vi "Autonomous Independent.vi"() -> ()   [LabVIEW 2015]
doc: "This VI is called when autonomous begins, and will automatically be terminated when autonomous ends. You can carry out timed or sensor driven robot movement independently without needing to return to the caller."
uses:
  <vilib>/Analysis/coordinate.llb/2D Cartesian Coordinate Rotation (Scalar).vi
  <vilib>/Analysis/coordinate.llb/2D Cartesian Coordinate Shift (Array).vi
  <vilib>/Rock Robotics/WPI/Utilities/WPI_GetSetVariantRefNum.vi
  <vilib>/Rock Robotics/Network Tables/SD Write Numeric Array.vi
  <vilib>/addons/control/pid/pid.llb/PID (DBL).vi
  <vilib>/Rock Robotics/WPI/RobotDrive/WPI_RobotDriveMecanumDrive_Polar.vi
  <vilib>/Analysis/NI_AALPro.lvlib
  <vilib>/addons/control/pid/NI_PID_pid.lvlib
  <vilib>/Rock Robotics/Network Tables/SD Read Number.vi
  <vilib>/Rock Robotics/WPI/RobotDrive/WPI_RobotDriveMecanumDrive_Cartesian.vi
panel:
  out "Y Out":dbl[](array[numeric])
  out "X Out":dbl[](array[numeric])
  out "Current Movement, for debugging":T1 {"Z Joystick Value" scale=-1.0..1.0; "Y Joystick Value" scale=1.0..-1.0; "X Joystick Value" scale=-1.0..1.0}
  in  "Array of robot movements":T2(array[cluster]) {"Z Joystick Value" scale=-1.0..1.0; "Y Joystick Value" scale=1.0..-1.0; "X Joystick Value" scale=-1.0..1.0}
  # "Be sure to right-click and choose Data Operations>>Make Current Value default if you want to save the array values with the VI"
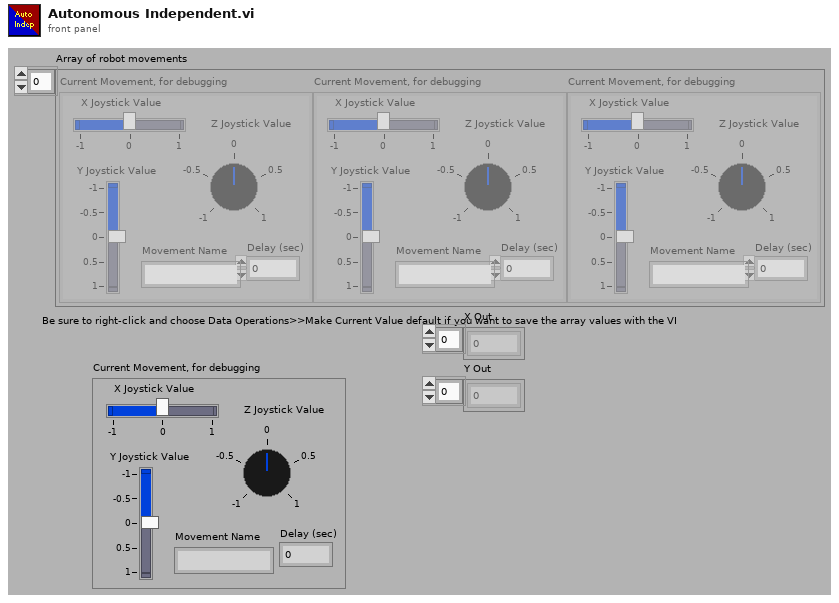
[diagram p1: front panel]
types:
  T1 = cluster{"X Joystick Value":dbl, "Y Joystick Value":dbl, "Z Joystick Value":dbl, "Delay (sec)":dbl, "Movement Name":string}
  T2 = cluster{"X Joystick Value":dbl, "Y Joystick Value":dbl, "Z Joystick Value":dbl, "Delay (sec)":dbl, "Movement Name":string}[]
  T3 = enum16{"Bin In", "Move Back", "Move Right", "Push Forward", "Stop"}
  T4 = typedef "WPI_JoystickDevRef.ctl" = cluster{"Device":T5}
  T5 = typedef "WPI_JoystickDeviceEnum.ctl" = enum16{"USB 0", "USB 1", "USB 2", "USB 3", "USB 4", "USB 5"}
  T6 = enum16{"Bin In", "Bin Up", "Tote In", "Move Sideways", "Advance", "Turn", "Dive Forward"}
  T7 = cluster{"proportional gain (Kc)":dbl, "integral time (Ti, min)":dbl, "derivative time (Td, min)":dbl}
  T8 = typedef "WPI_RobotDriveDevRef.ctl" = cluster{"DevStatus":errorcluster, "Motors[]":T9[], "Square Inputs":bool, "Max Output":dbl}
  T9 = typedef "WPI_MotorControlDeviceRef.ctl" = cluster{"DeviceStatus":errorcluster, "Type":T10, "PWM":cluster{"PWM Channel":T11, "DeadBand":T12}, "CAN":cluster{"Device Number":u8, "Control Mode":T13, "Semaphore":T14, "Max Vout":dbl, "TalonSRX Control Mode":T15}, "Invert":bool}
  T10 = typedef "WPI_MotorControlType.ctl" = enum16{"PWM", "CAN", "CANTalonSRX"}
  T11 = typedef "FPGA_DIOPWMChannel.ctl" = enum8{"PWM 0", "PWM 1", "PWM 2", "PWM 3", "PWM 4", "PWM 5", "PWM 6", "PWM 7", "PWM 8", "PWM 9", "PWM MXP 0", "PWM MXP 1", "PWM MXP 2", "PWM MXP 3", "PWM MXP 4", "PWM MXP 5", "PWM MXP 6", "PWM MXP 7", "PWM MXP 8", "PWM MXP 9", "Invalid"}
  T12 = typedef "WPI_PWMDeadband.ctl" = cluster{"Name":string, "maxPositivePwm":i32, "minPositivePwm":i32, "centerPwm":i32, "maxNegativePwm":i32, "minNegativePwm":i32, "angularRange":u16}
  T13 = typedef "WPI_CANJaguar_ControlMode.ctl" = enum8{"Percent VBus", "Current", "Speed", "Position", "Voltage"}
  T14 = typedef "Semaphore RefNum" = refnum<k1>
  T15 = typedef "WPI_CANTalonSRX_APIControlMode.ctl" = enum8{"Percent VBus", "Speed", "Position", "Slave", "Unchanged / Invalid", "Voltage Compensation", "Current", "Motion Profile"}
  T16 = typedef "WPI_GyroDevRef.ctl" = cluster{"DevStatus":errorcluster, "Analog Channel":T17, "Offset":dbl, "Gain (VoltsPerDegree/Second)":dbl, "Gyro Type":enum16{"Analog", "XRS450"}, "Handle":i32, "SPI Bus":T18, "Device Found":bool, "Sample Rate":dbl, "Calibrate On Open":bool}
  T17 = typedef "FPGA_AIChannel.ctl" = enum8{"AI 0", "AI 1", "AI 2", "AI 3", "AI MXP 0", "AI MXP 1", "AI MXP 2", "AI MXP 3", "Invalid"}
  T18 = typedef "spi_bus.ctl" = enum16{"SPI On-Board, CS0", "SPI On-Board, CS1", "SPI On-Board, CS2", "SPI On-Board, CS3", "SPI MXP", "Invalid"}
  T19 = typedef "WPI_DigitalInputDevRef.ctl" = cluster{"DevStatus":errorcluster, "DIO Channel":T20}
  T20 = typedef "FPGA_DIOChannel.ctl" = enum8{"DIO 0", "DIO 1", "DIO 2", "DIO 3", "DIO 4", "DIO 5", "DIO 6", "DIO 7", "DIO 8", "DIO 9", "DIO MXP 0", "DIO MXP 1", "DIO MXP 2", "DIO MXP 3", "DIO MXP 4", "DIO MXP 5", "DIO MXP 6", "DIO MXP 7", "DIO MXP 8", "DIO MXP 9", "DIO MXP 10", "DIO MXP 11", "DIO MXP 12", "DIO MXP 13", "DIO MXP 14", "DIO MXP 15", "Invalid"}
  T21 = typedef "WPI_AccelerometerDevRef.ctl" = cluster{"DevStatus":errorcluster, "Scaling":T22, "Analog Channels":T23, "I2C Bus":T24, "SPI Bus":T18, "Accel Range":T25, "ADXL Axes":T26, "Handle":i32, "Device Address":u8, "Accel Type":enum16{"Analog", "ADXL345 I2C", "ADXL345 SPI", "Internal", "ADXL362 SPI"}}
  T22 = typedef "WPI_AccelerometerScaling.ctl" = cluster{"Gain (VoltsPerG)":dbl, "Center Voltage":dbl}
  T23 = typedef "WPI_AccelerometerAnalogChannels.ctl" = cluster{"X-Axis":T17, "Y-Axis":T17, "Z-Axis":T17}
  T24 = typedef "i2c_bus.ctl" = enum16{"I2C On-Board", "I2C MXP", "Invalid"}
  T25 = typedef "ADXL345 Range.ctl" = u8
  T26 = typedef "WPI_AccelerometerADXL345 Axes.ctl" = cluster{"X-Axis":bool, "Y-Axis":bool, "Z-Axis":bool}
  T27 = cluster{"X-Axis":dbl, "Y-Axis":dbl, "Z-Axis":dbl}
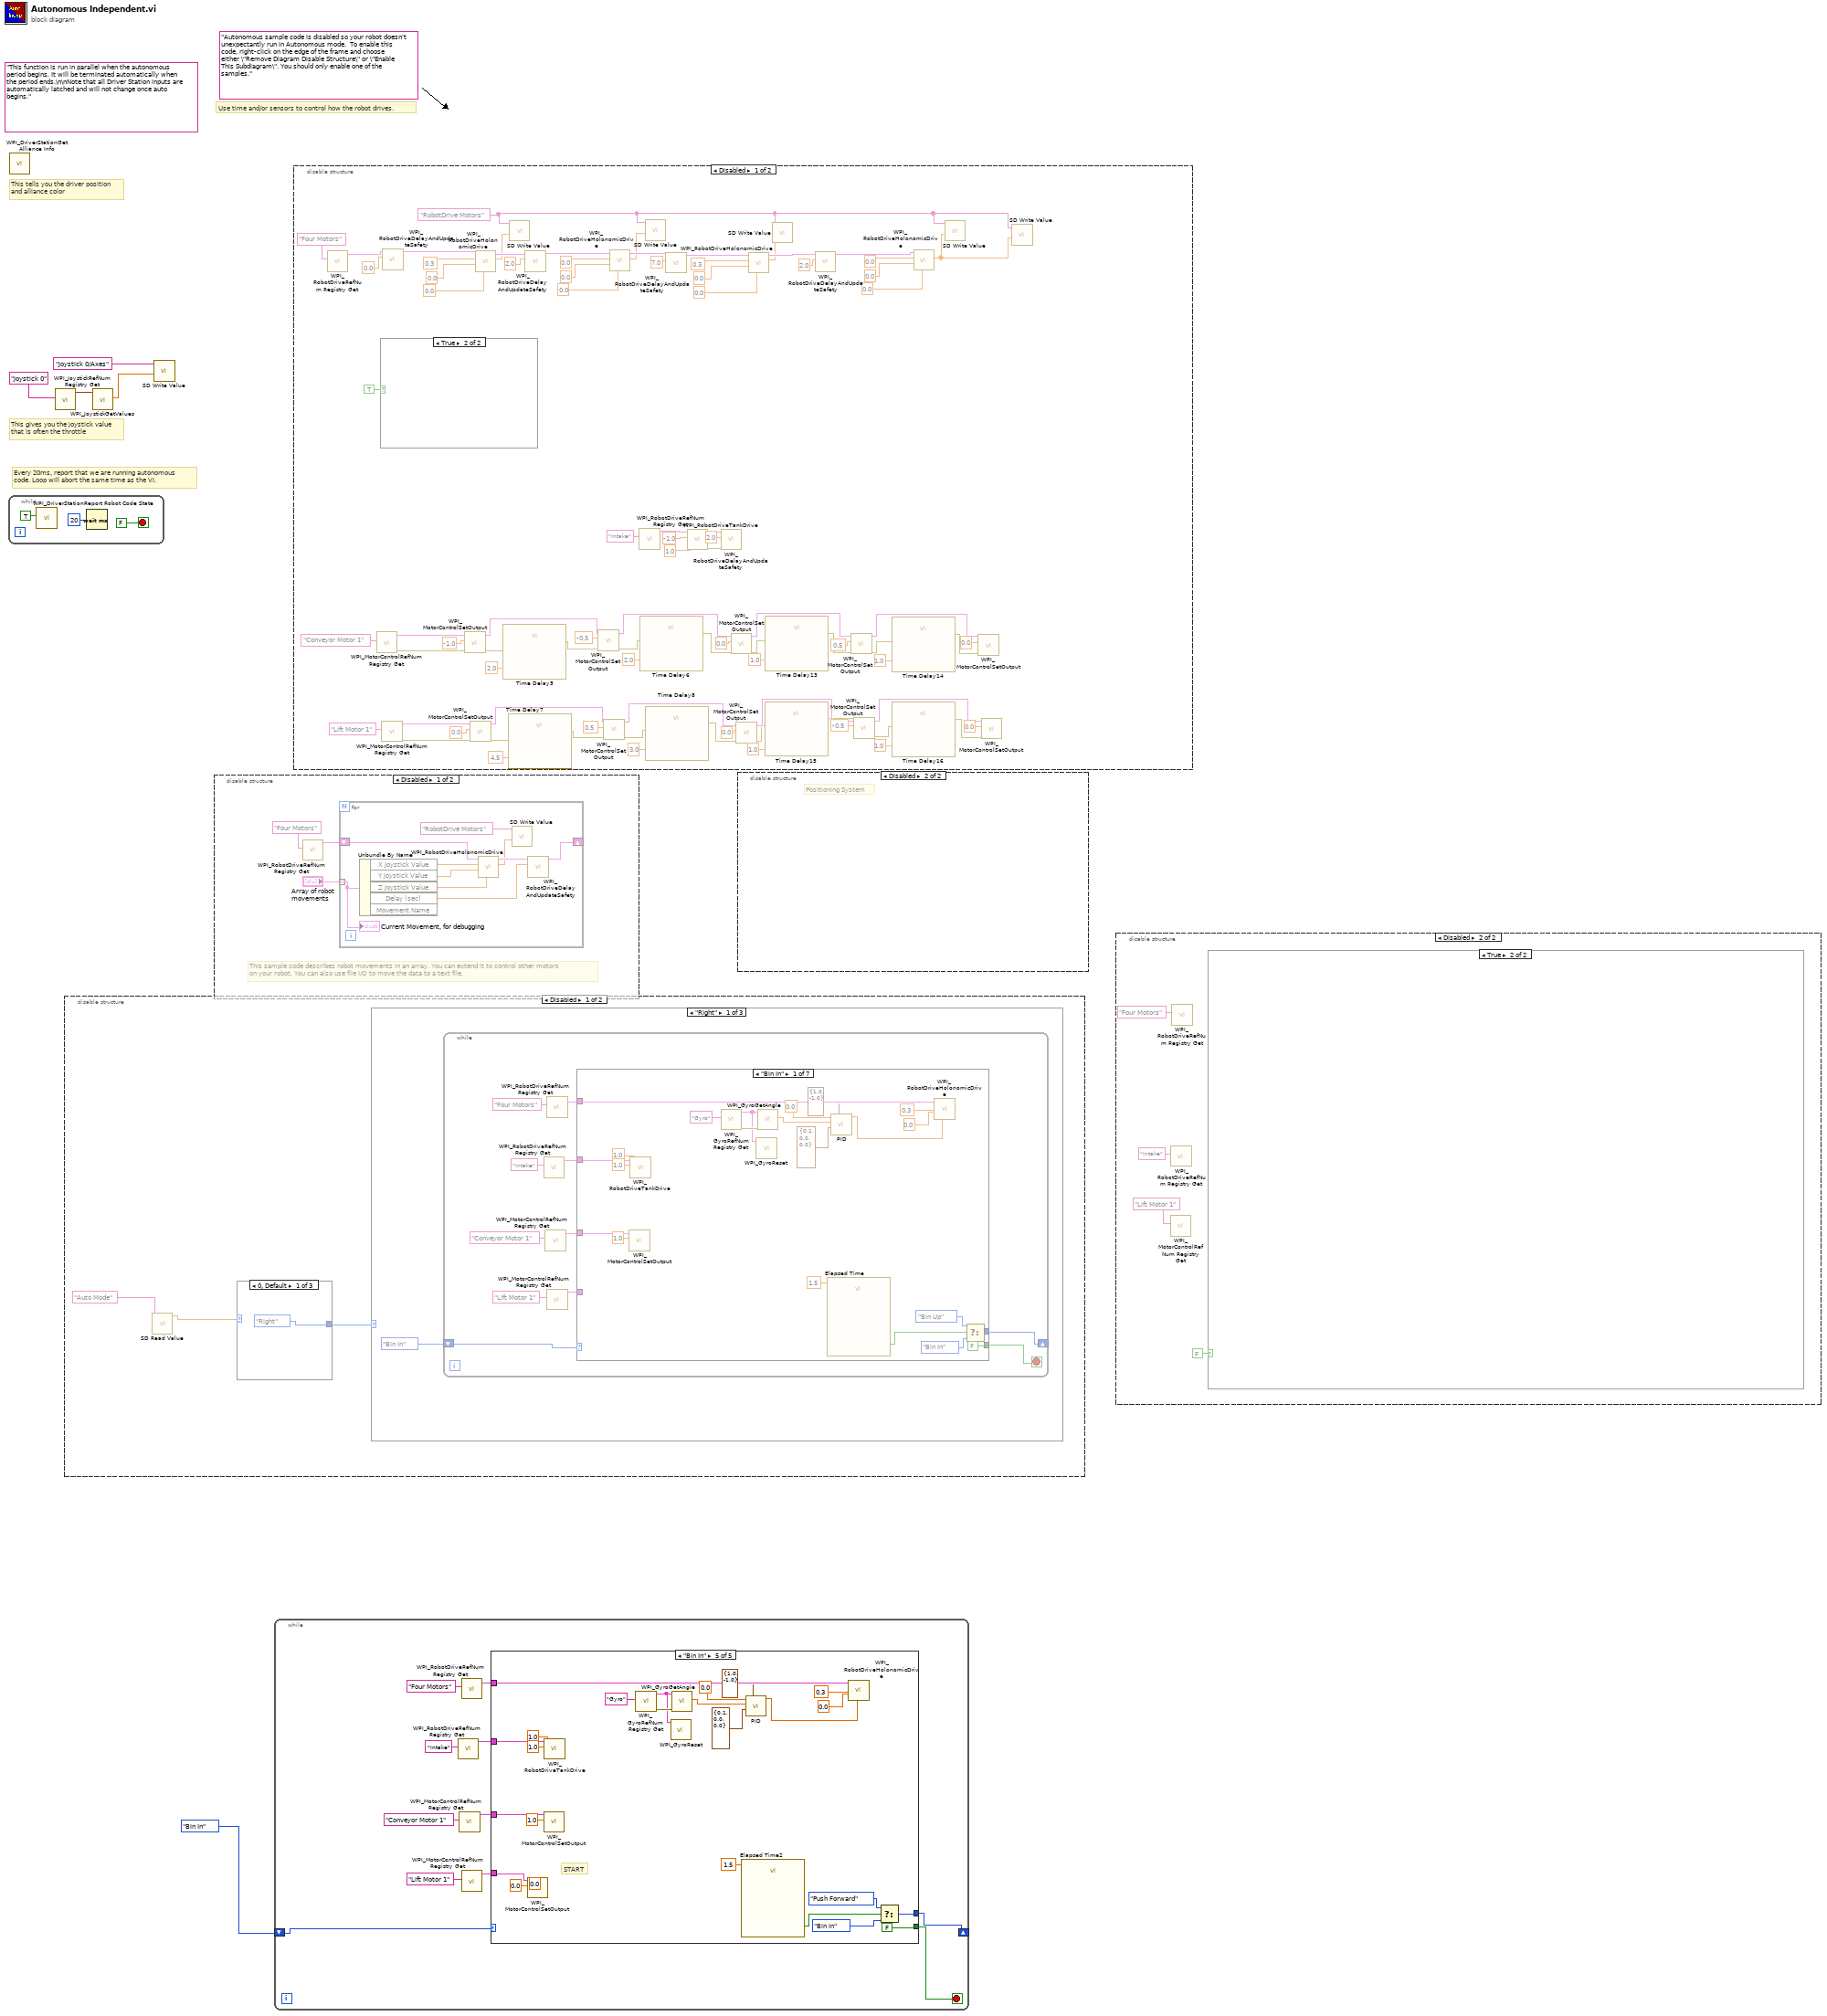
[diagram p0: block diagram]
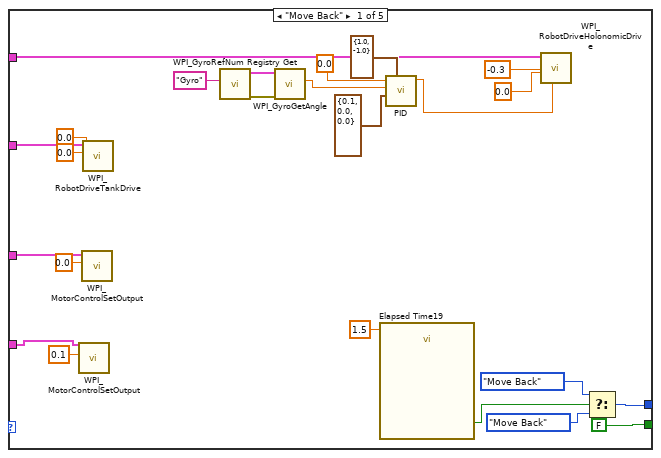
[diagram p2: hidden frame]
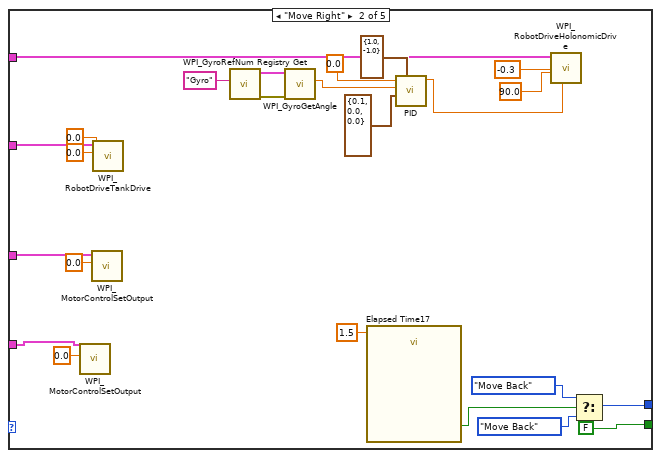
[diagram p3: hidden frame]
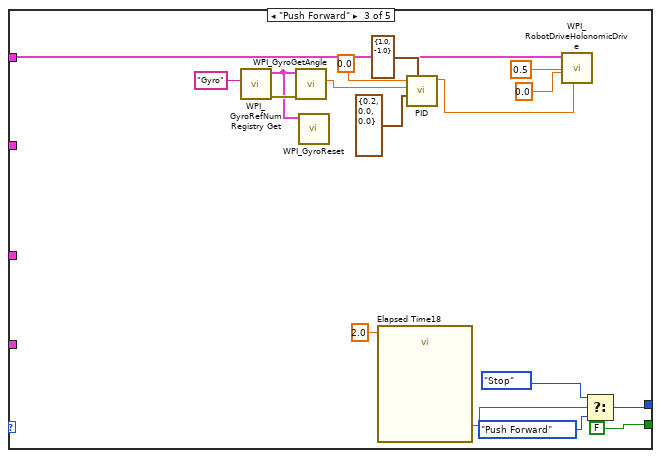
[diagram p4: hidden frame]
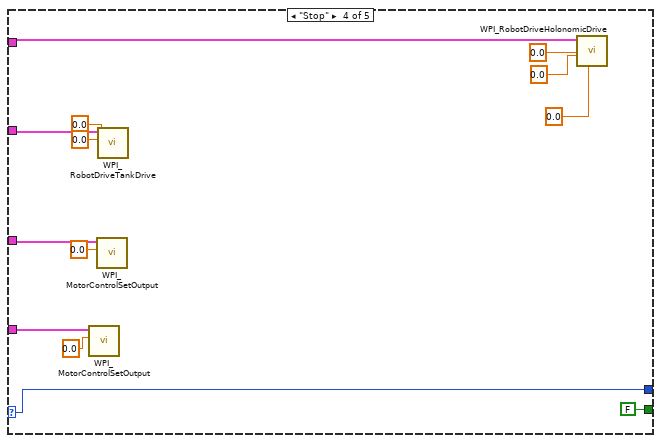
[diagram p5: hidden frame]
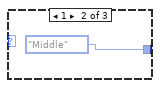
[diagram p6: hidden frame]
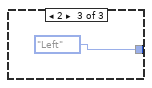
[diagram p7: hidden frame]
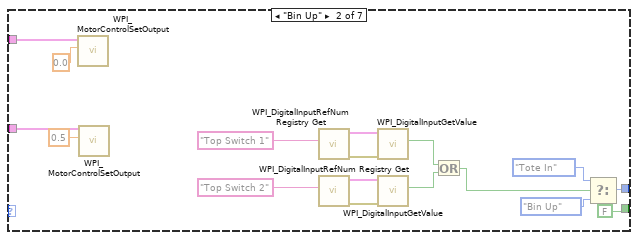
[diagram p8: hidden frame]
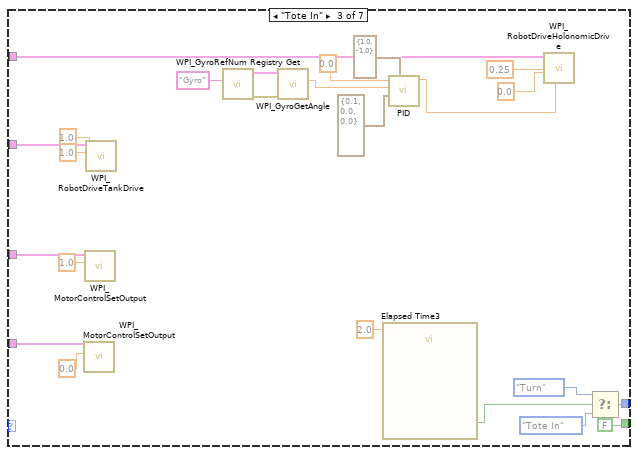
[diagram p9: hidden frame]
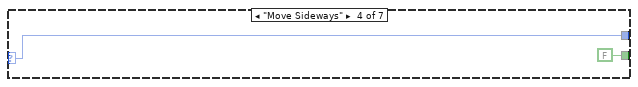
[diagram p10: hidden frame]
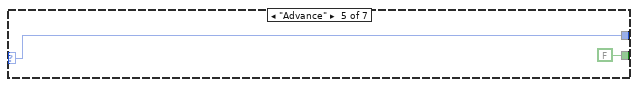
[diagram p11: hidden frame]
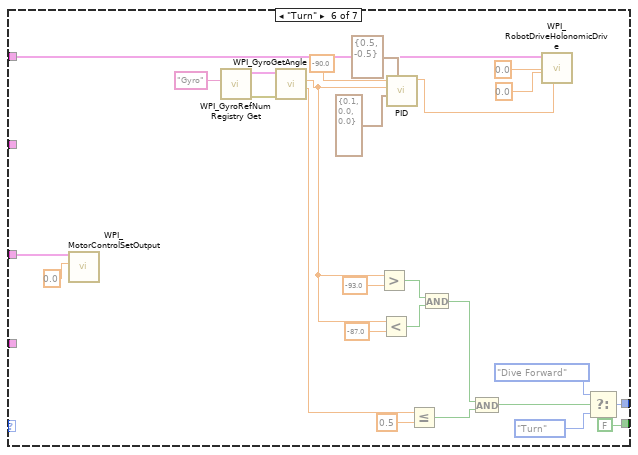
[diagram p12: hidden frame]
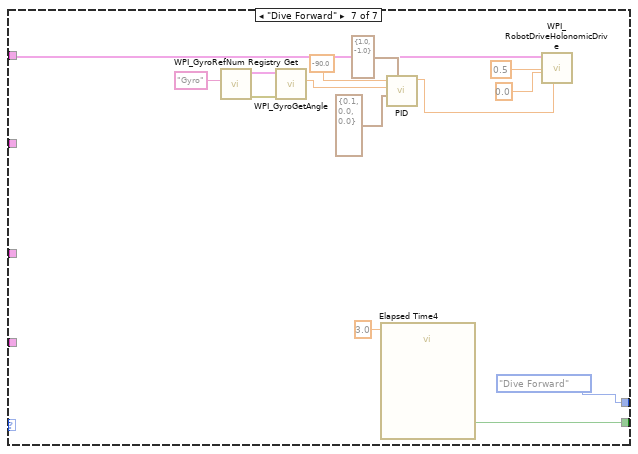
[diagram p13: hidden frame]
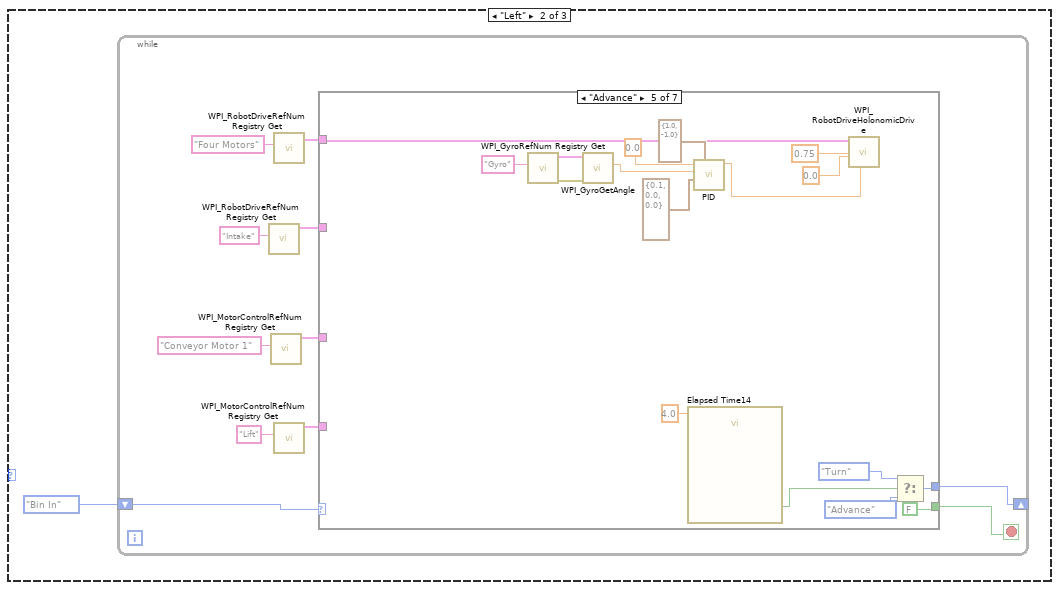
[diagram p14: hidden frame]
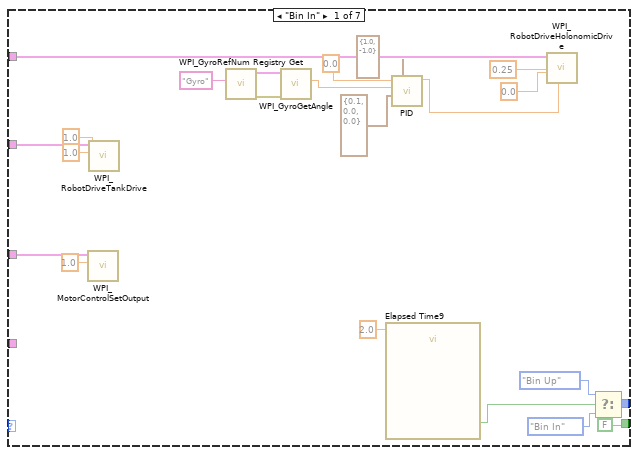
[diagram p15: hidden frame]
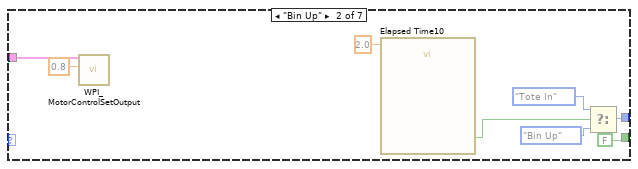
[diagram p16: hidden frame]
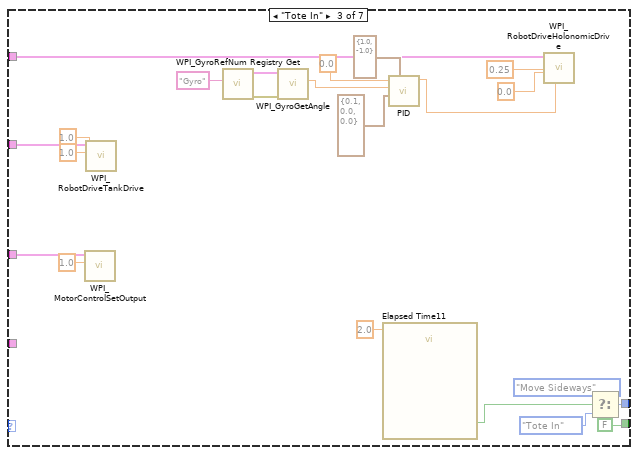
[diagram p17: hidden frame]
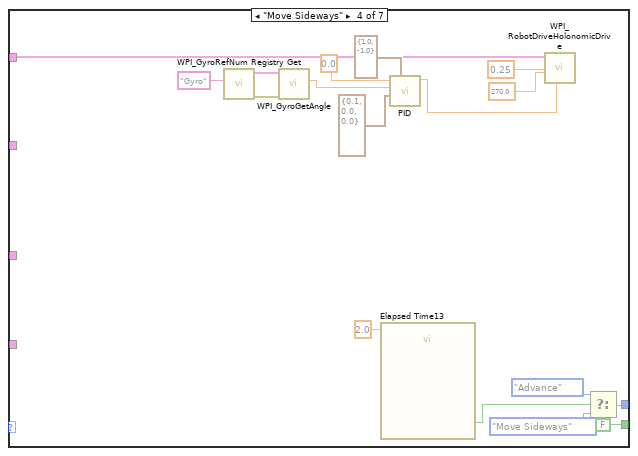
[diagram p18: hidden frame]
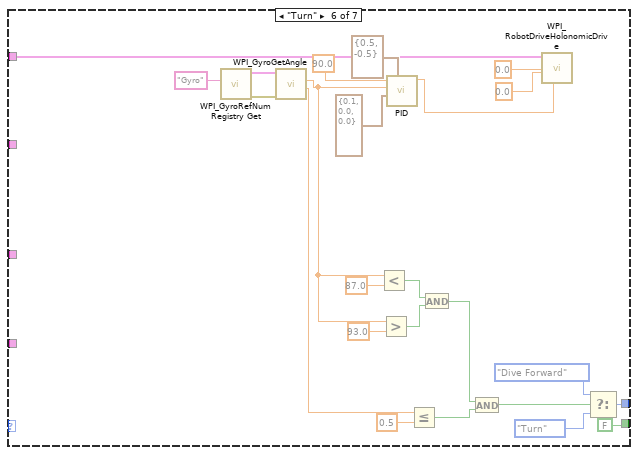
[diagram p19: hidden frame]
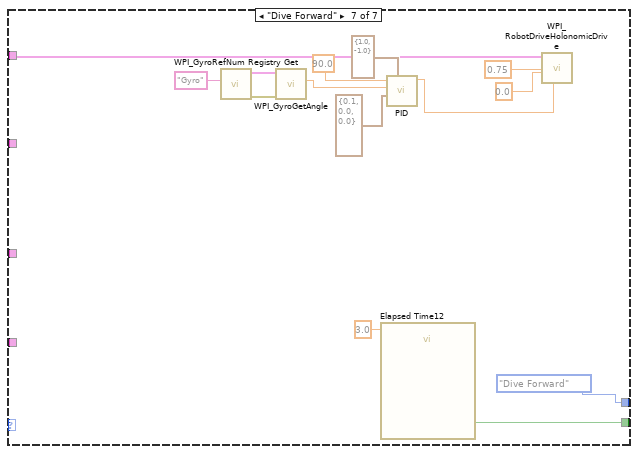
[diagram p20: hidden frame]
diagram:
  (unwired) "Autonomous sample code is disabled so your robot doesn't unexpectantly run in Autonomous mode.  To enable this code, right-click on the edge of the frame and choose either \"Remove Diagram Disable Structure\" or \"Enable This Subdiagram\". You should only enable one of the samples."
  (unwired) "This function is run in parallel when the autonomous period begins. It will be terminated automatically when the period ends.\n\nNote that all Driver Station inputs are automatically latched and will not change once auto begins."
  # "Every 20ms, report that we are running autonomous\ncode. Loop will abort the same time as the VI."
  # "This gives you the joystick value\nthat is often the throttle"
  # "Use time and/or sensors to control how the robot drives."
  # "This tells you the driver position\nand alliance color"
  n1 = while {
    stop <- FALSE stop-if-true
    n2 = call <vilib>:"WPI_DriverStationReport Robot Code State.vi"("Autonomous"=TRUE) -> ()  [unwired: 10 in, 1 out]
    n3 = Wait (ms)(milliseconds to wait=u32 20) -> ()  [unwired: 1 out]
  }
  n4 = call <vilib>:"WPI_DriverStationGet Alliance Info.vi"() -> ()  [unwired: 12 out]
  n5 = call <vilib>:"WPI_JoystickRefNum Registry Get.vi"("refnum name"="Joystick 0") -> ("JoystickDevRef"=w4:T4)  [unwired: 1 in, 9 out]
  n6 = disable-structure shown="Disabled" {
    frame Disabled {
      n7 = call-poly <vilib>:"SD Read Value.vi"("Name"="Auto Mode") -> ("Numeric"=w11:dbl)  [unwired: 8 in, 2 out]
      n8 = case shown="0, Default" w11 {
        tunnel: [enum16{"Left", "Middle", "Right"}."Right" enum16{"Left", "Middle", "Right"}."Middle" enum16{"Left", "Middle", "Right"}."Left"] -> w10
        frame 0, Default {
        }
        frame 1 {
        }
        frame 2 {
        }
      }
      n9 = case shown="\"Right\"" w10 {
        frame "Right" {
          n10 = while {
            shift-right: [w20] -> _
            shift-left: T6."Bin In" -> [w26]
            stop <- w16 stop-if-true
            n11 = call <vilib>:"WPI_RobotDriveRefNum Registry Get.vi"("refnum name"="Intake") -> ("RobotDriveDevRef"=w19:T8)  [unwired: 9 in, 1 out]
            n12 = call <vilib>:"WPI_MotorControlRefNum Registry Get.vi"("refnum name"="Conveyor Motor 1") -> ("MotorControlDevRef"=w18:T9)  [unwired: 9 in, 1 out]
            n13 = call <vilib>:"WPI_RobotDriveRefNum Registry Get.vi"("refnum name"="Four Motors") -> ("RobotDriveDevRef"=w21:T8)  [unwired: 9 in, 1 out]
            n14 = call <vilib>:"WPI_MotorControlRefNum Registry Get.vi"("refnum name"="Lift Motor 1") -> ("MotorControlDevRef"=w17:T9)  [unwired: 9 in, 1 out]
            n15 = case shown="\"Bin In\"" w26 {
              selector: w26 -> [_ _ _ w91 w93 _ _]
              tunnel: w21 -> [w48 _ w72 _ _ w109 w122]
              tunnel: [w38 w63 w71 w91 w93 w110 T6."Dive Forward"] -> w20
              tunnel: w19 -> [w37 _ w73 _ _ _ _]
              tunnel: w18 -> [w36 w58 w74 _ _ w94 _]
              tunnel: w17 -> [_ w65 w66 _ _ _ _]
              tunnel: [FALSE ("Time has Elapsed") FALSE ("Time has Elapsed") FALSE ("Time has Elapsed") FALSE ("Time has Elapsed") FALSE ("Time has Elapsed") FALSE ("Time has Elapsed") w120] -> w16
              frame "Bin In" {
                n16 = call <vilib>:"WPI_MotorControlSetOutput.vi"("Output"=1.0, "MotorControlDevRef"=w36) -> ()  [unwired: 7 in, 3 out]
                n17 = call <vilib>:"WPI_RobotDriveTankDrive.vi"("Right axis value"=1.0, "Left axis value"=1.0, "RobotDriveDevRef"=w37) -> ()  [unwired: 6 in, 3 out]
                n18 = call <vilib>:"WPI_GyroRefNum Registry Get.vi"("refnum name"="Gyro") -> ("error out"=w42:errorcluster, "GyroDevRef"=w27:T16)  [unwired: 9 in]
                n19 = call <vilib>:"WPI_GyroReset.vi"("GyroDevRef"=w27) -> ()  [unwired: 9 in, 2 out]
                n20 = call <vilib>:"WPI_GyroGetAngle.vi"("error in"=w42, "GyroDevRef"=w27) -> ("Angle"=w41:dbl)  [unwired: 5 in, 4 out]
                n21 = call "Elapsed Time"("Time Target (s)"=1.5) -> ("Time has Elapsed"=w31:bool)  [unwired: 11 in, 7 out]
                n22 = call-poly <vilib>:"PID.vi"("output range"=cluster{"output high":dbl, "output low":dbl} {"output high"=1.0, "output low"=-1.0}, "PID gains"=T7 {"proportional gain (Kc)"=0.1, "integral time (Ti, min)"=0.0, "derivative time (Td, min)"=0.0}, "process variable"=w41, "setpoint"=0.0) -> ("output"=w39:dbl)  [unwired: 6 in, 1 out]
                n23 = call-poly <vilib>:"WPI_RobotDriveHolonomicDrive.vi"("Rotation"=w39, "Direction"=0.0, "Magnitude"=0.3, "RobotDriveDevRef"=w48) -> ()  [unwired: 5 in, 3 out]
                n24 = Select(t=T6."Bin Up", s=w31, f=T6."Bin In") -> (s? t:f=w38:T6)
              }
              frame "Bin Up" {
                n25 = call <vilib>:"WPI_MotorControlSetOutput.vi"("Output"=0.0, "MotorControlDevRef"=w58) -> ()  [unwired: 7 in, 3 out]
                n26 = call <vilib>:"WPI_MotorControlSetOutput.vi"("Output"=0.5, "MotorControlDevRef"=w65) -> ()  [unwired: 7 in, 3 out]
                n27 = call <vilib>:"WPI_DigitalInputRefNum Registry Get.vi"("refnum name"="Top Switch 1") -> ("error out"=w56:errorcluster, "DigitalInputDevRef"=w55:T19)  [unwired: 9 in]
                n28 = call <vilib>:"WPI_DigitalInputRefNum Registry Get.vi"("refnum name"="Top Switch 2") -> ("error out"=w53:errorcluster, "DigitalInputDevRef"=w52:T19)  [unwired: 9 in]
                n29 = call <vilib>:"WPI_DigitalInputGetValue.vi"("error in (no error)"=w56, "DigitalInputDevRef"=w55) -> ("Value"=w51:bool)  [unwired: 7 in, 2 out]
                n30 = call <vilib>:"WPI_DigitalInputGetValue.vi"("error in (no error)"=w53, "DigitalInputDevRef"=w52) -> ("Value"=w50:bool)  [unwired: 7 in, 2 out]
                n31 = Or(x=w51, y=w50) -> (x .or. y?=w49:bool)
                n32 = Select(t=T6."Tote In", s=w49, f=T6."Bin Up") -> (s? t:f=w63:T6)
              }
              frame "Tote In" {
                n33 = call <vilib>:"WPI_MotorControlSetOutput.vi"("Output"=0.0, "MotorControlDevRef"=w66) -> ()  [unwired: 7 in, 3 out]
                n34 = call <vilib>:"WPI_MotorControlSetOutput.vi"("Output"=1.0, "MotorControlDevRef"=w74) -> ()  [unwired: 7 in, 3 out]
                n35 = call <vilib>:"WPI_RobotDriveTankDrive.vi"("Right axis value"=1.0, "Left axis value"=1.0, "RobotDriveDevRef"=w73) -> ()  [unwired: 6 in, 3 out]
                n36 = call <vilib>:"WPI_GyroRefNum Registry Get.vi"("refnum name"="Gyro") -> ("error out"=w80:errorcluster, "GyroDevRef"=w81:T16)  [unwired: 9 in]
                n37 = call <vilib>:"WPI_GyroGetAngle.vi"("error in"=w80, "GyroDevRef"=w81) -> ("Angle"=w82:dbl)  [unwired: 5 in, 4 out]
                n38 = call "Elapsed Time3"("Time Target (s)"=2.0) -> ("Time has Elapsed"=w89:bool)  [unwired: 11 in, 7 out]
                n39 = call-poly <vilib>:"PID.vi"("output range"=cluster{"output high":dbl, "output low":dbl} {"output high"=1.0, "output low"=-1.0}, "PID gains"=T7 {"proportional gain (Kc)"=0.1, "integral time (Ti, min)"=0.0, "derivative time (Td, min)"=0.0}, "process variable"=w82, "setpoint"=0.0) -> ("output"=w84:dbl)  [unwired: 6 in, 1 out]
                n40 = call-poly <vilib>:"WPI_RobotDriveHolonomicDrive.vi"("Rotation"=w84, "Direction"=0.0, "Magnitude"=0.25, "RobotDriveDevRef"=w72) -> ()  [unwired: 5 in, 3 out]
                n41 = Select(t=T6."Turn", s=w89, f=T6."Tote In") -> (s? t:f=w71:T6)
              }
              frame "Move Sideways" {
              }
              frame "Advance" {
              }
              frame "Turn" {
                n42 = call <vilib>:"WPI_MotorControlSetOutput.vi"("Output"=0.0, "MotorControlDevRef"=w94) -> ()  [unwired: 7 in, 3 out]
                n43 = call <vilib>:"WPI_GyroRefNum Registry Get.vi"("refnum name"="Gyro") -> ("error out"=w114:errorcluster, "GyroDevRef"=w113:T16)  [unwired: 9 in]
                n44 = call <vilib>:"WPI_GyroGetAngle.vi"("error in"=w114, "GyroDevRef"=w113) -> ("Angular Rate"=w108:dbl, "Angle"=w106:dbl)  [unwired: 5 in, 3 out]
                n45 = Greater?(x=w106, y=-93.0) -> (0:w103:bool)
                n46 = Less?(x=w106, y=-87.0) -> (x < y?=w102:bool)
                n47 = call-poly <vilib>:"PID.vi"("output range"=cluster{"output high":dbl, "output low":dbl} {"output high"=0.5, "output low"=-0.5}, "PID gains"=T7 {"proportional gain (Kc)"=0.1, "integral time (Ti, min)"=0.0, "derivative time (Td, min)"=0.0}, "process variable"=w106, "setpoint"=-90.0) -> ("output"=w111:dbl)  [unwired: 6 in, 1 out]
                n48 = Less Or Equal?(x=w108, y=0.5) -> (x <= y?=w101:bool)
                n49 = And(x=w103, y=w102) -> (x .and. y?=w100:bool)
                n50 = And(x=w100, y=w101) -> (x .and. y?=w99:bool)
                n51 = call-poly <vilib>:"WPI_RobotDriveHolonomicDrive.vi"("Rotation"=w111, "Direction"=0.0, "Magnitude"=0.0, "RobotDriveDevRef"=w109) -> ()  [unwired: 5 in, 3 out]
                n52 = Select(t=T6."Dive Forward", s=w99, f=T6."Turn") -> (s? t:f=w110:T6)
              }
              frame "Dive Forward" {
                n53 = call <vilib>:"WPI_GyroRefNum Registry Get.vi"("refnum name"="Gyro") -> ("error out"=w128:errorcluster, "GyroDevRef"=w129:T16)  [unwired: 9 in]
                n54 = call <vilib>:"WPI_GyroGetAngle.vi"("error in"=w128, "GyroDevRef"=w129) -> ("Angle"=w130:dbl)  [unwired: 5 in, 4 out]
                n55 = call "Elapsed Time4"("Time Target (s)"=3.0) -> ("Time has Elapsed"=w120:bool)  [unwired: 11 in, 7 out]
                n56 = call-poly <vilib>:"PID.vi"("output range"=cluster{"output high":dbl, "output low":dbl} {"output high"=1.0, "output low"=-1.0}, "PID gains"=T7 {"proportional gain (Kc)"=0.1, "integral time (Ti, min)"=0.0, "derivative time (Td, min)"=0.0}, "process variable"=w130, "setpoint"=-90.0) -> ("output"=w132:dbl)  [unwired: 6 in, 1 out]
                n57 = call-poly <vilib>:"WPI_RobotDriveHolonomicDrive.vi"("Rotation"=w132, "Direction"=0.0, "Magnitude"=0.5, "RobotDriveDevRef"=w122) -> ()  [unwired: 5 in, 3 out]
              }
            }
          }
        }
        frame "Left" {
          n58 = while {
            shift-right: [w139] -> _
            shift-left: T6."Bin In" -> [w145]
            stop <- w135 stop-if-true
            n59 = call <vilib>:"WPI_RobotDriveRefNum Registry Get.vi"("refnum name"="Intake") -> ("RobotDriveDevRef"=w138:T8)  [unwired: 9 in, 1 out]
            n60 = call <vilib>:"WPI_MotorControlRefNum Registry Get.vi"("refnum name"="Conveyor Motor 1") -> ("MotorControlDevRef"=w137:T9)  [unwired: 9 in, 1 out]
            n61 = call <vilib>:"WPI_RobotDriveRefNum Registry Get.vi"("refnum name"="Four Motors") -> ("RobotDriveDevRef"=w140:T8)  [unwired: 9 in, 1 out]
            n62 = call <vilib>:"WPI_MotorControlRefNum Registry Get.vi"("refnum name"="Lift") -> ("MotorControlDevRef"=w136:T9)  [unwired: 9 in, 1 out]
            n63 = case shown="\"Advance\"" w145 {
              tunnel: w140 -> [w167 _ w180 w200 w217 w245 w258]
              tunnel: [w156 w171 w179 w199 w216 w246 T6."Dive Forward"] -> w139
              tunnel: w138 -> [w155 _ w181 _ _ _ _]
              tunnel: w137 -> [w154 _ w182 _ _ _ _]
              tunnel: w136 -> [_ w175 _ _ _ _ _]
              tunnel: [FALSE ("Time has Elapsed") FALSE ("Time has Elapsed") FALSE ("Time has Elapsed") FALSE ("Time has Elapsed") FALSE ("Time has Elapsed") FALSE ("Time has Elapsed") w256] -> w135
              frame "Bin In" {
                n64 = call <vilib>:"WPI_MotorControlSetOutput.vi"("Output"=1.0, "MotorControlDevRef"=w154) -> ()  [unwired: 7 in, 3 out]
                n65 = call <vilib>:"WPI_RobotDriveTankDrive.vi"("Right axis value"=1.0, "Left axis value"=1.0, "RobotDriveDevRef"=w155) -> ()  [unwired: 6 in, 3 out]
                n66 = call <vilib>:"WPI_GyroRefNum Registry Get.vi"("refnum name"="Gyro") -> ("error out"=w161:errorcluster, "GyroDevRef"=w160:T16)  [unwired: 9 in]
                n67 = call <vilib>:"WPI_GyroGetAngle.vi"("error in"=w161, "GyroDevRef"=w160) -> ("Angle"=w159:dbl)  [unwired: 5 in, 4 out]
                n68 = call "Elapsed Time9"("Time Target (s)"=2.0) -> ("Time has Elapsed"=w149:bool)  [unwired: 11 in, 7 out]
                n69 = call-poly <vilib>:"PID.vi"("output range"=cluster{"output high":dbl, "output low":dbl} {"output high"=1.0, "output low"=-1.0}, "PID gains"=T7 {"proportional gain (Kc)"=0.1, "integral time (Ti, min)"=0.0, "derivative time (Td, min)"=0.0}, "process variable"=w159, "setpoint"=0.0) -> ("output"=w157:dbl)  [unwired: 6 in, 1 out]
                n70 = call-poly <vilib>:"WPI_RobotDriveHolonomicDrive.vi"("Rotation"=w157, "Direction"=0.0, "Magnitude"=0.25, "RobotDriveDevRef"=w167) -> ()  [unwired: 5 in, 3 out]
                n71 = Select(t=T6."Bin Up", s=w149, f=T6."Bin In") -> (s? t:f=w156:T6)
              }
              frame "Bin Up" {
                n72 = call <vilib>:"WPI_MotorControlSetOutput.vi"("Output"=0.8, "MotorControlDevRef"=w175) -> ()  [unwired: 7 in, 3 out]
                n73 = call "Elapsed Time10"("Time Target (s)"=2.0) -> ("Time has Elapsed"=w173:bool)  [unwired: 11 in, 7 out]
                n74 = Select(t=T6."Tote In", s=w173, f=T6."Bin Up") -> (s? t:f=w171:T6)
              }
              frame "Tote In" {
                n75 = call <vilib>:"WPI_MotorControlSetOutput.vi"("Output"=1.0, "MotorControlDevRef"=w182) -> ()  [unwired: 7 in, 3 out]
                n76 = call <vilib>:"WPI_RobotDriveTankDrive.vi"("Right axis value"=1.0, "Left axis value"=1.0, "RobotDriveDevRef"=w181) -> ()  [unwired: 6 in, 3 out]
                n77 = call <vilib>:"WPI_GyroRefNum Registry Get.vi"("refnum name"="Gyro") -> ("error out"=w188:errorcluster, "GyroDevRef"=w189:T16)  [unwired: 9 in]
                n78 = call <vilib>:"WPI_GyroGetAngle.vi"("error in"=w188, "GyroDevRef"=w189) -> ("Angle"=w190:dbl)  [unwired: 5 in, 4 out]
                n79 = call "Elapsed Time11"("Time Target (s)"=2.0) -> ("Time has Elapsed"=w197:bool)  [unwired: 11 in, 7 out]
                n80 = call-poly <vilib>:"PID.vi"("output range"=cluster{"output high":dbl, "output low":dbl} {"output high"=1.0, "output low"=-1.0}, "PID gains"=T7 {"proportional gain (Kc)"=0.1, "integral time (Ti, min)"=0.0, "derivative time (Td, min)"=0.0}, "process variable"=w190, "setpoint"=0.0) -> ("output"=w192:dbl)  [unwired: 6 in, 1 out]
                n81 = call-poly <vilib>:"WPI_RobotDriveHolonomicDrive.vi"("Rotation"=w192, "Direction"=0.0, "Magnitude"=0.25, "RobotDriveDevRef"=w180) -> ()  [unwired: 5 in, 3 out]
                n82 = Select(t=T6."Move Sideways", s=w197, f=T6."Tote In") -> (s? t:f=w179:T6)
              }
              frame "Move Sideways" {
                n83 = call <vilib>:"WPI_GyroRefNum Registry Get.vi"("refnum name"="Gyro") -> ("error out"=w208:errorcluster, "GyroDevRef"=w209:T16)  [unwired: 9 in]
                n84 = call <vilib>:"WPI_GyroGetAngle.vi"("error in"=w208, "GyroDevRef"=w209) -> ("Angle"=w210:dbl)  [unwired: 5 in, 4 out]
                n85 = call "Elapsed Time13"("Time Target (s)"=2.0) -> ("Time has Elapsed"=w214:bool)  [unwired: 11 in, 7 out]
                n86 = call-poly <vilib>:"PID.vi"("output range"=cluster{"output high":dbl, "output low":dbl} {"output high"=1.0, "output low"=-1.0}, "PID gains"=T7 {"proportional gain (Kc)"=0.1, "integral time (Ti, min)"=0.0, "derivative time (Td, min)"=0.0}, "process variable"=w210, "setpoint"=0.0) -> ("output"=w212:dbl)  [unwired: 6 in, 1 out]
                n87 = call-poly <vilib>:"WPI_RobotDriveHolonomicDrive.vi"("Rotation"=w212, "Direction"=270.0, "Magnitude"=0.25, "RobotDriveDevRef"=w200) -> ()  [unwired: 5 in, 3 out]
                n88 = Select(t=T6."Advance", s=w214, f=T6."Move Sideways") -> (s? t:f=w199:T6)
              }
              frame "Advance" {
                n89 = call <vilib>:"WPI_GyroRefNum Registry Get.vi"("refnum name"="Gyro") -> ("error out"=w225:errorcluster, "GyroDevRef"=w226:T16)  [unwired: 9 in]
                n90 = call <vilib>:"WPI_GyroGetAngle.vi"("error in"=w225, "GyroDevRef"=w226) -> ("Angle"=w227:dbl)  [unwired: 5 in, 4 out]
                n91 = call "Elapsed Time14"("Time Target (s)"=4.0) -> ("Time has Elapsed"=w231:bool)  [unwired: 11 in, 7 out]
                n92 = call-poly <vilib>:"PID.vi"("output range"=cluster{"output high":dbl, "output low":dbl} {"output high"=1.0, "output low"=-1.0}, "PID gains"=T7 {"proportional gain (Kc)"=0.1, "integral time (Ti, min)"=0.0, "derivative time (Td, min)"=0.0}, "process variable"=w227, "setpoint"=0.0) -> ("output"=w229:dbl)  [unwired: 6 in, 1 out]
                n93 = call-poly <vilib>:"WPI_RobotDriveHolonomicDrive.vi"("Rotation"=w229, "Direction"=0.0, "Magnitude"=0.75, "RobotDriveDevRef"=w217) -> ()  [unwired: 5 in, 3 out]
                n94 = Select(t=T6."Turn", s=w231, f=T6."Advance") -> (s? t:f=w216:T6)
              }
              frame "Turn" {
                n95 = call <vilib>:"WPI_GyroRefNum Registry Get.vi"("refnum name"="Gyro") -> ("error out"=w250:errorcluster, "GyroDevRef"=w249:T16)  [unwired: 9 in]
                n96 = call <vilib>:"WPI_GyroGetAngle.vi"("error in"=w250, "GyroDevRef"=w249) -> ("Angular Rate"=w244:dbl, "Angle"=w242:dbl)  [unwired: 5 in, 3 out]
                n97 = Less?(x=w242, y=87.0) -> (x < y?=w239:bool)
                n98 = Greater?(x=w242, y=93.0) -> (0:w238:bool)
                n99 = call-poly <vilib>:"PID.vi"("output range"=cluster{"output high":dbl, "output low":dbl} {"output high"=0.5, "output low"=-0.5}, "PID gains"=T7 {"proportional gain (Kc)"=0.1, "integral time (Ti, min)"=0.0, "derivative time (Td, min)"=0.0}, "process variable"=w242, "setpoint"=90.0) -> ("output"=w247:dbl)  [unwired: 6 in, 1 out]
                n100 = Less Or Equal?(x=w244, y=0.5) -> (x <= y?=w237:bool)
                n101 = And(x=w239, y=w238) -> (x .and. y?=w236:bool)
                n102 = And(x=w236, y=w237) -> (x .and. y?=w235:bool)
                n103 = call-poly <vilib>:"WPI_RobotDriveHolonomicDrive.vi"("Rotation"=w247, "Direction"=0.0, "Magnitude"=0.0, "RobotDriveDevRef"=w245) -> ()  [unwired: 5 in, 3 out]
                n104 = Select(t=T6."Dive Forward", s=w235, f=T6."Turn") -> (s? t:f=w246:T6)
              }
              frame "Dive Forward" {
                n105 = call <vilib>:"WPI_GyroRefNum Registry Get.vi"("refnum name"="Gyro") -> ("error out"=w264:errorcluster, "GyroDevRef"=w265:T16)  [unwired: 9 in]
                n106 = call <vilib>:"WPI_GyroGetAngle.vi"("error in"=w264, "GyroDevRef"=w265) -> ("Angle"=w266:dbl)  [unwired: 5 in, 4 out]
                n107 = call "Elapsed Time12"("Time Target (s)"=3.0) -> ("Time has Elapsed"=w256:bool)  [unwired: 11 in, 7 out]
                n108 = call-poly <vilib>:"PID.vi"("output range"=cluster{"output high":dbl, "output low":dbl} {"output high"=1.0, "output low"=-1.0}, "PID gains"=T7 {"proportional gain (Kc)"=0.1, "integral time (Ti, min)"=0.0, "derivative time (Td, min)"=0.0}, "process variable"=w266, "setpoint"=90.0) -> ("output"=w268:dbl)  [unwired: 6 in, 1 out]
                n109 = call-poly <vilib>:"WPI_RobotDriveHolonomicDrive.vi"("Rotation"=w268, "Direction"=0.0, "Magnitude"=0.75, "RobotDriveDevRef"=w258) -> ()  [unwired: 5 in, 3 out]
              }
            }
          }
        }
        frame "Middle" {
          n110 = while {
            shift-right: [w275] -> _
            shift-left: T6."Bin In" -> [w281]
            stop <- w271 stop-if-true
            n111 = call <vilib>:"WPI_RobotDriveRefNum Registry Get.vi"("refnum name"="Intake") -> ("RobotDriveDevRef"=w274:T8)  [unwired: 9 in, 1 out]
            n112 = call <vilib>:"WPI_MotorControlRefNum Registry Get.vi"("refnum name"="Conveyor Motor 1") -> ("MotorControlDevRef"=w273:T9)  [unwired: 9 in, 1 out]
            n113 = call <vilib>:"WPI_RobotDriveRefNum Registry Get.vi"("refnum name"="Four Motors") -> ("RobotDriveDevRef"=w276:T8)  [unwired: 9 in, 1 out]
            n114 = call <vilib>:"WPI_MotorControlRefNum Registry Get.vi"("refnum name"="Lift") -> ("MotorControlDevRef"=w272:T9)  [unwired: 9 in, 1 out]
            n115 = case shown="\"Advance\"" w281 {
              tunnel: w276 -> [w303 _ w316 w336 w353 w381 w394]
              tunnel: [w292 w307 w315 w335 w352 w382 T6."Dive Forward"] -> w275
              tunnel: w274 -> [w291 _ w317 _ _ _ _]
              tunnel: w273 -> [w290 _ w318 _ _ _ _]
              tunnel: w272 -> [_ w311 _ _ _ _ _]
              tunnel: [FALSE ("Time has Elapsed") FALSE ("Time has Elapsed") FALSE ("Time has Elapsed") FALSE ("Time has Elapsed") FALSE ("Time has Elapsed") FALSE ("Time has Elapsed") w392] -> w271
              frame "Bin In" {
                n116 = call <vilib>:"WPI_MotorControlSetOutput.vi"("Output"=1.0, "MotorControlDevRef"=w290) -> ()  [unwired: 7 in, 3 out]
                n117 = call <vilib>:"WPI_RobotDriveTankDrive.vi"("Right axis value"=1.0, "Left axis value"=1.0, "RobotDriveDevRef"=w291) -> ()  [unwired: 6 in, 3 out]
                n118 = call <vilib>:"WPI_GyroRefNum Registry Get.vi"("refnum name"="Gyro") -> ("error out"=w297:errorcluster, "GyroDevRef"=w296:T16)  [unwired: 9 in]
                n119 = call <vilib>:"WPI_GyroGetAngle.vi"("error in"=w297, "GyroDevRef"=w296) -> ("Angle"=w295:dbl)  [unwired: 5 in, 4 out]
                n120 = call "Elapsed Time5"("Time Target (s)"=2.0) -> ("Time has Elapsed"=w285:bool)  [unwired: 11 in, 7 out]
                n121 = call-poly <vilib>:"PID.vi"("output range"=cluster{"output high":dbl, "output low":dbl} {"output high"=1.0, "output low"=-1.0}, "PID gains"=T7 {"proportional gain (Kc)"=0.1, "integral time (Ti, min)"=0.0, "derivative time (Td, min)"=0.0}, "process variable"=w295, "setpoint"=0.0) -> ("output"=w293:dbl)  [unwired: 6 in, 1 out]
                n122 = call-poly <vilib>:"WPI_RobotDriveHolonomicDrive.vi"("Rotation"=w293, "Direction"=0.0, "Magnitude"=0.25, "RobotDriveDevRef"=w303) -> ()  [unwired: 5 in, 3 out]
                n123 = Select(t=T6."Bin Up", s=w285, f=T6."Bin In") -> (s? t:f=w292:T6)
              }
              frame "Bin Up" {
                n124 = call <vilib>:"WPI_MotorControlSetOutput.vi"("Output"=0.8, "MotorControlDevRef"=w311) -> ()  [unwired: 7 in, 3 out]
                n125 = call "Elapsed Time6"("Time Target (s)"=2.0) -> ("Time has Elapsed"=w309:bool)  [unwired: 11 in, 7 out]
                n126 = Select(t=T6."Tote In", s=w309, f=T6."Bin Up") -> (s? t:f=w307:T6)
              }
              frame "Tote In" {
                n127 = call <vilib>:"WPI_MotorControlSetOutput.vi"("Output"=1.0, "MotorControlDevRef"=w318) -> ()  [unwired: 7 in, 3 out]
                n128 = call <vilib>:"WPI_RobotDriveTankDrive.vi"("Right axis value"=1.0, "Left axis value"=1.0, "RobotDriveDevRef"=w317) -> ()  [unwired: 6 in, 3 out]
                n129 = call <vilib>:"WPI_GyroRefNum Registry Get.vi"("refnum name"="Gyro") -> ("error out"=w324:errorcluster, "GyroDevRef"=w325:T16)  [unwired: 9 in]
                n130 = call <vilib>:"WPI_GyroGetAngle.vi"("error in"=w324, "GyroDevRef"=w325) -> ("Angle"=w326:dbl)  [unwired: 5 in, 4 out]
                n131 = call "Elapsed Time7"("Time Target (s)"=2.0) -> ("Time has Elapsed"=w333:bool)  [unwired: 11 in, 7 out]
                n132 = call-poly <vilib>:"PID.vi"("output range"=cluster{"output high":dbl, "output low":dbl} {"output high"=1.0, "output low"=-1.0}, "PID gains"=T7 {"proportional gain (Kc)"=0.1, "integral time (Ti, min)"=0.0, "derivative time (Td, min)"=0.0}, "process variable"=w326, "setpoint"=0.0) -> ("output"=w328:dbl)  [unwired: 6 in, 1 out]
                n133 = call-poly <vilib>:"WPI_RobotDriveHolonomicDrive.vi"("Rotation"=w328, "Direction"=0.0, "Magnitude"=0.25, "RobotDriveDevRef"=w316) -> ()  [unwired: 5 in, 3 out]
                n134 = Select(t=T6."Move Sideways", s=w333, f=T6."Tote In") -> (s? t:f=w315:T6)
              }
              frame "Move Sideways" {
                n135 = call <vilib>:"WPI_GyroRefNum Registry Get.vi"("refnum name"="Gyro") -> ("error out"=w344:errorcluster, "GyroDevRef"=w345:T16)  [unwired: 9 in]
                n136 = call <vilib>:"WPI_GyroGetAngle.vi"("error in"=w344, "GyroDevRef"=w345) -> ("Angle"=w346:dbl)  [unwired: 5 in, 4 out]
                n137 = call "Elapsed Time8"("Time Target (s)"=2.0) -> ("Time has Elapsed"=w350:bool)  [unwired: 11 in, 7 out]
                n138 = call-poly <vilib>:"PID.vi"("output range"=cluster{"output high":dbl, "output low":dbl} {"output high"=1.0, "output low"=-1.0}, "PID gains"=T7 {"proportional gain (Kc)"=0.1, "integral time (Ti, min)"=0.0, "derivative time (Td, min)"=0.0}, "process variable"=w346, "setpoint"=0.0) -> ("output"=w348:dbl)  [unwired: 6 in, 1 out]
                n139 = call-poly <vilib>:"WPI_RobotDriveHolonomicDrive.vi"("Rotation"=w348, "Direction"=270.0, "Magnitude"=0.25, "RobotDriveDevRef"=w336) -> ()  [unwired: 5 in, 3 out]
                n140 = Select(t=T6."Advance", s=w350, f=T6."Move Sideways") -> (s? t:f=w335:T6)
              }
              frame "Advance" {
                n141 = call <vilib>:"WPI_GyroRefNum Registry Get.vi"("refnum name"="Gyro") -> ("error out"=w361:errorcluster, "GyroDevRef"=w362:T16)  [unwired: 9 in]
                n142 = call <vilib>:"WPI_GyroGetAngle.vi"("error in"=w361, "GyroDevRef"=w362) -> ("Angle"=w363:dbl)  [unwired: 5 in, 4 out]
                n143 = call "Elapsed Time15"("Time Target (s)"=2.0) -> ("Time has Elapsed"=w367:bool)  [unwired: 11 in, 7 out]
                n144 = call-poly <vilib>:"PID.vi"("output range"=cluster{"output high":dbl, "output low":dbl} {"output high"=1.0, "output low"=-1.0}, "PID gains"=T7 {"proportional gain (Kc)"=0.1, "integral time (Ti, min)"=0.0, "derivative time (Td, min)"=0.0}, "process variable"=w363, "setpoint"=0.0) -> ("output"=w365:dbl)  [unwired: 6 in, 1 out]
                n145 = call-poly <vilib>:"WPI_RobotDriveHolonomicDrive.vi"("Rotation"=w365, "Direction"=0.0, "Magnitude"=0.75, "RobotDriveDevRef"=w353) -> ()  [unwired: 5 in, 3 out]
                n146 = Select(t=T6."Turn", s=w367, f=T6."Advance") -> (s? t:f=w352:T6)
              }
              frame "Turn" {
                n147 = call <vilib>:"WPI_GyroRefNum Registry Get.vi"("refnum name"="Gyro") -> ("error out"=w386:errorcluster, "GyroDevRef"=w385:T16)  [unwired: 9 in]
                n148 = call <vilib>:"WPI_GyroGetAngle.vi"("error in"=w386, "GyroDevRef"=w385) -> ("Angular Rate"=w380:dbl, "Angle"=w378:dbl)  [unwired: 5 in, 3 out]
                n149 = Less?(x=w378, y=87.0) -> (x < y?=w375:bool)
                n150 = Greater?(x=w378, y=93.0) -> (0:w374:bool)
                n151 = call-poly <vilib>:"PID.vi"("output range"=cluster{"output high":dbl, "output low":dbl} {"output high"=0.5, "output low"=-0.5}, "PID gains"=T7 {"proportional gain (Kc)"=0.1, "integral time (Ti, min)"=0.0, "derivative time (Td, min)"=0.0}, "process variable"=w378, "setpoint"=90.0) -> ("output"=w383:dbl)  [unwired: 6 in, 1 out]
                n152 = Less Or Equal?(x=w380, y=0.5) -> (x <= y?=w373:bool)
                n153 = And(x=w375, y=w374) -> (x .and. y?=w372:bool)
                n154 = And(x=w372, y=w373) -> (x .and. y?=w371:bool)
                n155 = call-poly <vilib>:"WPI_RobotDriveHolonomicDrive.vi"("Rotation"=w383, "Direction"=0.0, "Magnitude"=0.0, "RobotDriveDevRef"=w381) -> ()  [unwired: 5 in, 3 out]
                n156 = Select(t=T6."Dive Forward", s=w371, f=T6."Turn") -> (s? t:f=w382:T6)
              }
              frame "Dive Forward" {
                n157 = call <vilib>:"WPI_GyroRefNum Registry Get.vi"("refnum name"="Gyro") -> ("error out"=w400:errorcluster, "GyroDevRef"=w401:T16)  [unwired: 9 in]
                n158 = call <vilib>:"WPI_GyroGetAngle.vi"("error in"=w400, "GyroDevRef"=w401) -> ("Angle"=w402:dbl)  [unwired: 5 in, 4 out]
                n159 = call "Elapsed Time16"("Time Target (s)"=3.0) -> ("Time has Elapsed"=w392:bool)  [unwired: 11 in, 7 out]
                n160 = call-poly <vilib>:"PID.vi"("output range"=cluster{"output high":dbl, "output low":dbl} {"output high"=1.0, "output low"=-1.0}, "PID gains"=T7 {"proportional gain (Kc)"=0.1, "integral time (Ti, min)"=0.0, "derivative time (Td, min)"=0.0}, "process variable"=w402, "setpoint"=90.0) -> ("output"=w404:dbl)  [unwired: 6 in, 1 out]
                n161 = call-poly <vilib>:"WPI_RobotDriveHolonomicDrive.vi"("Rotation"=w404, "Direction"=0.0, "Magnitude"=0.75, "RobotDriveDevRef"=w394) -> ()  [unwired: 5 in, 3 out]
              }
            }
          }
        }
      }
    }
    frame Enabled {
    }
  }
  n162 = call <vilib>:"WPI_JoystickGetValues.vi"("JoystickDevRef"=w4) -> ("Axes"=w2:dbl[])  [unwired: 6 in, 4 out]
  n163 = call-poly <vilib>:"SD Write Value.vi"("Numeric Array"=w2, "Name"="Joystick 0/Axes") -> ()  [unwired: 8 in, 2 out]
  n164 = disable-structure shown="Disabled" {
    frame Disabled {
      # "This sample code describes robot movements in an array. You can extend it to control other motors\non your robot. You can also use file I/O to move the data to a text file."
      n165 = call <vilib>:"WPI_RobotDriveRefNum Registry Get.vi"("refnum name"="Four Motors") -> ("RobotDriveDevRef"=w407:T8)  [unwired: 1 in, 9 out]
      n166 = for {
        shift-right: [w415] -> _
        shift-left: w407 -> [w416]
        tunnel: "Array of robot movements" -> [w411] mode=indexing
        n167 = Unbundle By Name(w411) -> ("X Joystick Value"=w414:dbl, "Y Joystick Value"=w413:dbl, "Z Joystick Value"=w410:dbl, "Delay (sec)"=w412:dbl)  [unwired: 1 out]
        n168 = call-poly <vilib>:"WPI_RobotDriveHolonomicDrive.vi"("Rotation"=w410, "Y"=w413, "X"=w414, "RobotDriveDevRef"=w416) -> ("Motor Values"=w409:dbl[], "RobotDriveDevRef"=w417:T8)  [unwired: 5 in, 1 out]
        n169 = call-poly <vilib>:"SD Write Value.vi"("Numeric Array"=w409, "Name"="RobotDrive Motors") -> ()  [unwired: 8 in, 2 out]
        n170 = call <vilib>:"WPI_RobotDriveDelayAndUpdateSafety.vi"("Delay (s)"=w412, "RobotDriveDevRef"=w417) -> ("RobotDriveDevRef 2"=w415:T8)  [unwired: 8 in, 1 out]
        "Current Movement, for debugging" <- w411
      }
    }
    frame Enabled {
    }
  }
  n171 = while {
    shift-right: [w420] -> _
    shift-left: T3."Bin In" -> [w421]
    stop <- w419 stop-if-true
    n172 = call <vilib>:"WPI_RobotDriveRefNum Registry Get.vi"("refnum name"="Intake") -> ("RobotDriveDevRef"=w424:T8)  [unwired: 9 in, 1 out]
    n173 = call <vilib>:"WPI_MotorControlRefNum Registry Get.vi"("refnum name"="Conveyor Motor 1") -> ("MotorControlDevRef"=w423:T9)  [unwired: 9 in, 1 out]
    n174 = call <vilib>:"WPI_RobotDriveRefNum Registry Get.vi"("refnum name"="Four Motors") -> ("RobotDriveDevRef"=w425:T8)  [unwired: 9 in, 1 out]
    n175 = call <vilib>:"WPI_MotorControlRefNum Registry Get.vi"("refnum name"="Lift Motor 1") -> ("MotorControlDevRef"=w422:T9)  [unwired: 9 in, 1 out]
    n176 = case shown="\"Bin In\"" w421 {
      selector: w421 -> [_ _ _ w504 _]
      tunnel: w425 -> [w436 w460 w480 w505 w531]
      tunnel: [w433 w459 w482 w504 w521] -> w420
      tunnel: w424 -> [w435 w461 _ w497 w520]
      tunnel: w423 -> [w434 w462 _ w498 w519]
      tunnel: w422 -> [w430 w454 _ w495 w508]
      tunnel: [FALSE ("Time has Elapsed") FALSE ("Time has Elapsed") FALSE ("Time has Elapsed") FALSE ("Time has Elapsed") FALSE ("Time has Elapsed")] -> w419
      frame "Move Back" {
        n177 = call <vilib>:"WPI_MotorControlSetOutput.vi"("Output"=0.1, "MotorControlDevRef"=w430) -> ()  [unwired: 7 in, 3 out]
        n178 = call <vilib>:"WPI_MotorControlSetOutput.vi"("Output"=0.0, "MotorControlDevRef"=w434) -> ()  [unwired: 7 in, 3 out]
        n179 = call <vilib>:"WPI_RobotDriveTankDrive.vi"("Right axis value"=0.0, "Left axis value"=0.0, "RobotDriveDevRef"=w435) -> ()  [unwired: 6 in, 3 out]
        n180 = call <vilib>:"WPI_GyroRefNum Registry Get.vi"("refnum name"="Gyro") -> ("error out"=w442:errorcluster, "GyroDevRef"=w451:T16)  [unwired: 9 in]
        n181 = call <vilib>:"WPI_GyroGetAngle.vi"("error in"=w442, "GyroDevRef"=w451) -> ("Angle"=w443:dbl)  [unwired: 5 in, 4 out]
        n182 = call "Elapsed Time19"("Time Target (s)"=1.5) -> ("Time has Elapsed"=w450:bool)  [unwired: 11 in, 7 out]
        n183 = call-poly <vilib>:"PID.vi"("output range"=cluster{"output high":dbl, "output low":dbl} {"output high"=1.0, "output low"=-1.0}, "PID gains"=T7 {"proportional gain (Kc)"=0.1, "integral time (Ti, min)"=0.0, "derivative time (Td, min)"=0.0}, "process variable"=w443, "setpoint"=0.0) -> ("output"=w445:dbl)  [unwired: 6 in, 1 out]
        n184 = call-poly <vilib>:"WPI_RobotDriveHolonomicDrive.vi"("Rotation"=w445, "Direction"=0.0, "Magnitude"=-0.3, "RobotDriveDevRef"=w436) -> ()  [unwired: 5 in, 3 out]
        n185 = Select(t=T3."Move Back", s=w450, f=T3."Move Back") -> (s? t:f=w433:T3)
      }
      frame "Move Right" {
        n186 = call <vilib>:"WPI_MotorControlSetOutput.vi"("Output"=0.0, "MotorControlDevRef"=w454) -> ()  [unwired: 7 in, 3 out]
        n187 = call <vilib>:"WPI_MotorControlSetOutput.vi"("Output"=0.0, "MotorControlDevRef"=w462) -> ()  [unwired: 7 in, 3 out]
        n188 = call <vilib>:"WPI_RobotDriveTankDrive.vi"("Right axis value"=0.0, "Left axis value"=0.0, "RobotDriveDevRef"=w461) -> ()  [unwired: 6 in, 3 out]
        n189 = call <vilib>:"WPI_GyroRefNum Registry Get.vi"("refnum name"="Gyro") -> ("error out"=w468:errorcluster, "GyroDevRef"=w477:T16)  [unwired: 9 in]
        n190 = call <vilib>:"WPI_GyroGetAngle.vi"("error in"=w468, "GyroDevRef"=w477) -> ("Angle"=w469:dbl)  [unwired: 5 in, 4 out]
        n191 = call "Elapsed Time17"("Time Target (s)"=1.5) -> ("Time has Elapsed"=w476:bool)  [unwired: 11 in, 7 out]
        n192 = call-poly <vilib>:"PID.vi"("output range"=cluster{"output high":dbl, "output low":dbl} {"output high"=1.0, "output low"=-1.0}, "PID gains"=T7 {"proportional gain (Kc)"=0.1, "integral time (Ti, min)"=0.0, "derivative time (Td, min)"=0.0}, "process variable"=w469, "setpoint"=0.0) -> ("output"=w471:dbl)  [unwired: 6 in, 1 out]
        n193 = call-poly <vilib>:"WPI_RobotDriveHolonomicDrive.vi"("Rotation"=w471, "Direction"=90.0, "Magnitude"=-0.3, "RobotDriveDevRef"=w460) -> ()  [unwired: 5 in, 3 out]
        n194 = Select(t=T3."Move Back", s=w476, f=T3."Move Back") -> (s? t:f=w459:T3)
      }
      frame "Push Forward" {
        n195 = call <vilib>:"WPI_GyroRefNum Registry Get.vi"("refnum name"="Gyro") -> ("error out"=w488:errorcluster, "GyroDevRef"=w478:T16)  [unwired: 9 in]
        n196 = call <vilib>:"WPI_GyroGetAngle.vi"("error in"=w488, "GyroDevRef"=w478) -> ("Angle"=w487:dbl)  [unwired: 5 in, 4 out]
        n197 = call <vilib>:"WPI_GyroReset.vi"("GyroDevRef"=w478) -> ()  [unwired: 9 in, 2 out]
        n198 = call "Elapsed Time18"("Time Target (s)"=2.0) -> ("Time has Elapsed"=w483:bool)  [unwired: 11 in, 7 out]
        n199 = call-poly <vilib>:"PID.vi"("output range"=cluster{"output high":dbl, "output low":dbl} {"output high"=1.0, "output low"=-1.0}, "PID gains"=T7 {"proportional gain (Kc)"=0.2, "integral time (Ti, min)"=0.0, "derivative time (Td, min)"=0.0}, "process variable"=w487, "setpoint"=0.0) -> ("output"=w485:dbl)  [unwired: 6 in, 1 out]
        n200 = call-poly <vilib>:"WPI_RobotDriveHolonomicDrive.vi"("Rotation"=w485, "Direction"=0.0, "Magnitude"=0.5, "RobotDriveDevRef"=w480) -> ()  [unwired: 5 in, 3 out]
        n201 = Select(t=T3."Stop", s=w483, f=T3."Push Forward") -> (s? t:f=w482:T3)
      }
      frame "Stop" {
        n202 = call <vilib>:"WPI_MotorControlSetOutput.vi"("Output"=0.0, "MotorControlDevRef"=w495) -> ()  [unwired: 7 in, 3 out]
        n203 = call <vilib>:"WPI_MotorControlSetOutput.vi"("Output"=0.0, "MotorControlDevRef"=w498) -> ()  [unwired: 7 in, 3 out]
        n204 = call <vilib>:"WPI_RobotDriveTankDrive.vi"("Right axis value"=0.0, "Left axis value"=0.0, "RobotDriveDevRef"=w497) -> ()  [unwired: 6 in, 3 out]
        n205 = call-poly <vilib>:"WPI_RobotDriveHolonomicDrive.vi"("Rotation"=0.0, "Direction"=0.0, "Magnitude"=0.0, "RobotDriveDevRef"=w505) -> ()  [unwired: 5 in, 3 out]
      }
      frame "Bin In" {
        (unwired) 0.0 ("Output")
        # "START"
        n206 = call <vilib>:"WPI_MotorControlSetOutput.vi"("Output"=0.0, "MotorControlDevRef"=w508) -> ()  [unwired: 7 in, 3 out]
        n207 = call <vilib>:"WPI_MotorControlSetOutput.vi"("Output"=1.0, "MotorControlDevRef"=w519) -> ()  [unwired: 7 in, 3 out]
        n208 = call <vilib>:"WPI_RobotDriveTankDrive.vi"("Right axis value"=1.0, "Left axis value"=1.0, "RobotDriveDevRef"=w520) -> ()  [unwired: 6 in, 3 out]
        n209 = call <vilib>:"WPI_GyroRefNum Registry Get.vi"("refnum name"="Gyro") -> ("error out"=w525:errorcluster, "GyroDevRef"=w512:T16)  [unwired: 9 in]
        n210 = call <vilib>:"WPI_GyroReset.vi"("GyroDevRef"=w512) -> ()  [unwired: 9 in, 2 out]
        n211 = call <vilib>:"WPI_GyroGetAngle.vi"("error in"=w525, "GyroDevRef"=w512) -> ("Angle"=w524:dbl)  [unwired: 5 in, 4 out]
        n212 = call "Elapsed Time2"("Time Target (s)"=1.5) -> ("Time has Elapsed"=w514:bool)  [unwired: 11 in, 7 out]
        n213 = call-poly <vilib>:"PID.vi"("output range"=cluster{"output high":dbl, "output low":dbl} {"output high"=1.0, "output low"=-1.0}, "PID gains"=T7 {"proportional gain (Kc)"=0.1, "integral time (Ti, min)"=0.0, "derivative time (Td, min)"=0.0}, "process variable"=w524, "setpoint"=0.0) -> ("output"=w522:dbl)  [unwired: 6 in, 1 out]
        n214 = call-poly <vilib>:"WPI_RobotDriveHolonomicDrive.vi"("Rotation"=w522, "Direction"=0.0, "Magnitude"=0.3, "RobotDriveDevRef"=w531) -> ()  [unwired: 5 in, 3 out]
        n215 = Select(t=T3."Push Forward", s=w514, f=T3."Bin In") -> (s? t:f=w521:T3)
      }
    }
  }
  n216 = disable-structure shown="Disabled" {
    frame Disabled {
      w565 = "RobotDrive Motors" ("Name")
      n217 = call <vilib>:"WPI_RobotDriveRefNum Registry Get.vi"("refnum name"="Four Motors") -> ("RobotDriveDevRef"=w595:T8)  [unwired: 1 in, 9 out]
      n218 = call <vilib>:"WPI_MotorControlRefNum Registry Get.vi"("refnum name"="Conveyor Motor 1") -> ("error out"=w585:errorcluster, "MotorControlDevRef"=w589:T9)  [unwired: 9 in]
      n219 = case shown="True" TRUE {
        frame False {
        }
        frame True {
        }
      }
      n220 = call <vilib>:"WPI_MotorControlRefNum Registry Get.vi"("refnum name"="Lift Motor 1") -> ("error out"=w573:errorcluster, "MotorControlDevRef"=w577:T9)  [unwired: 9 in]
      n221 = call <vilib>:"WPI_RobotDriveDelayAndUpdateSafety.vi"("Delay (s)"=0.0, "RobotDriveDevRef"=w595) -> ("RobotDriveDevRef 2"=w594:T8)  [unwired: 8 in, 1 out]
      n222 = call <vilib>:"WPI_MotorControlSetOutput.vi"("error in (no error)"=w585, "Output"=-1.0, "MotorControlDevRef"=w589) -> ("error out"=w586:errorcluster, "MotorControlDevRef"=w584:T9)  [unwired: 6 in, 1 out]
      n223 = call <vilib>:"WPI_MotorControlSetOutput.vi"("error in (no error)"=w573, "Output"=0.0, "MotorControlDevRef"=w577) -> ("error out"=w574:errorcluster, "MotorControlDevRef"=w572:T9)  [unwired: 6 in, 1 out]
      n224 = call-poly <vilib>:"WPI_RobotDriveHolonomicDrive.vi"("Rotation"=0.0, "Direction"=0.0 ("X axis value"), "Magnitude"=0.3 ("X axis value"), "RobotDriveDevRef"=w594) -> ("Motor Values"=w601:dbl[], "RobotDriveDevRef"=w611:T8)  [unwired: 5 in, 1 out]
      n225 = call "Time Delay5"("error in (no error)"=w586, "Delay Time (s)"=2.0) -> ("error out"=w583:errorcluster)  [unwired: 9 in]
      n226 = call "Time Delay7"("error in (no error)"=w574, "Delay Time (s)"=4.5) -> ("error out"=w571:errorcluster)  [unwired: 9 in]
      n227 = call-poly <vilib>:"SD Write Value.vi"("Numeric Array"=w601, "Name"=w565) -> ()  [unwired: 8 in, 2 out]
      n228 = call <vilib>:"WPI_RobotDriveDelayAndUpdateSafety.vi"("Delay (s)"=2.0, "RobotDriveDevRef"=w611) -> ("RobotDriveDevRef 2"=w610:T8)  [unwired: 8 in, 1 out]
      n229 = call <vilib>:"WPI_MotorControlSetOutput.vi"("error in (no error)"=w583, "Output"=-0.5, "MotorControlDevRef"=w584) -> ("error out"=w581:errorcluster, "MotorControlDevRef"=w580:T9)  [unwired: 6 in, 1 out]
      n230 = call <vilib>:"WPI_MotorControlSetOutput.vi"("error in (no error)"=w571, "Output"=0.5, "MotorControlDevRef"=w572) -> ("error out"=w569:errorcluster, "MotorControlDevRef"=w568:T9)  [unwired: 6 in, 1 out]
      n231 = call-poly <vilib>:"WPI_RobotDriveHolonomicDrive.vi"("Rotation"=0.0, "Direction"=0.0 ("X axis value"), "Magnitude"=0.0 ("X axis value"), "RobotDriveDevRef"=w610) -> ("Motor Values"=w600:dbl[], "RobotDriveDevRef"=w609:T8)  [unwired: 5 in, 1 out]
      n232 = call <vilib>:"WPI_RobotDriveRefNum Registry Get.vi"("refnum name"="Intake") -> ("RobotDriveDevRef"=w535:T8)  [unwired: 9 in, 1 out]
      n233 = call "Time Delay6"("error in (no error)"=w581, "Delay Time (s)"=2.0) -> ("error out"=w579:errorcluster)  [unwired: 9 in]
      n234 = call-poly <vilib>:"SD Write Value.vi"("Numeric Array"=w600, "Name"=w565) -> ()  [unwired: 8 in, 2 out]
      n235 = call "Time Delay8"("error in (no error)"=w569, "Delay Time (s)"=3.0) -> ("error out"=w567:errorcluster)  [unwired: 9 in]
      n236 = call <vilib>:"WPI_RobotDriveDelayAndUpdateSafety.vi"("Delay (s)"=7.0, "RobotDriveDevRef"=w609) -> ("RobotDriveDevRef 2"=w608:T8)  [unwired: 8 in, 1 out]
      n237 = call <vilib>:"WPI_RobotDriveTankDrive.vi"("Right axis value"=1.0, "Left axis value"=-1.0, "RobotDriveDevRef"=w535) -> ("error out"=w534:errorcluster, "RobotDriveDevRef"=w533:T8)  [unwired: 6 in, 1 out]
      n238 = call <vilib>:"WPI_RobotDriveDelayAndUpdateSafety.vi"("error in (no error)"=w534, "Delay (s)"=2.0, "RobotDriveDevRef"=w533) -> ()  [unwired: 7 in, 2 out]
      n239 = call <vilib>:"WPI_MotorControlSetOutput.vi"("error in (no error)"=w579, "Output"=0.0, "MotorControlDevRef"=w580) -> ("error out"=w561:errorcluster, "MotorControlDevRef"=w563:T9)  [unwired: 6 in, 1 out]
      n240 = call <vilib>:"WPI_MotorControlSetOutput.vi"("error in (no error)"=w567, "Output"=0.0, "MotorControlDevRef"=w568) -> ("error out"=w556:errorcluster, "MotorControlDevRef"=w557:T9)  [unwired: 6 in, 1 out]
      n241 = call-poly <vilib>:"WPI_RobotDriveHolonomicDrive.vi"("Rotation"=0.0 ("X axis value"), "Direction"=0.0 ("X axis value"), "Magnitude"=0.3 ("X axis value"), "RobotDriveDevRef"=w608) -> ("Motor Values"=w564:dbl[], "RobotDriveDevRef"=w592:T8)  [unwired: 5 in, 1 out]
      n242 = call "Time Delay15"("error in (no error)"=w556, "Delay Time (s)"=1.0) -> ("error out"=w555:errorcluster)  [unwired: 9 in]
      n243 = call "Time Delay13"("error in (no error)"=w561, "Delay Time (s)"=1.0) -> ("error out"=w560:errorcluster)  [unwired: 9 in]
      n244 = call-poly <vilib>:"SD Write Value.vi"("Numeric Array"=w564, "Name"=w565) -> ()  [unwired: 8 in, 2 out]
      n245 = call <vilib>:"WPI_RobotDriveDelayAndUpdateSafety.vi"("Delay (s)"=2.0, "RobotDriveDevRef"=w592) -> ("RobotDriveDevRef 2"=w591:T8)  [unwired: 8 in, 1 out]
      n246 = call <vilib>:"WPI_MotorControlSetOutput.vi"("error in (no error)"=w560, "Output"=0.5, "MotorControlDevRef"=w563) -> ("error out"=w559:errorcluster, "MotorControlDevRef"=w562:T9)  [unwired: 6 in, 1 out]
      n247 = call <vilib>:"WPI_MotorControlSetOutput.vi"("error in (no error)"=w555, "Output"=-0.5, "MotorControlDevRef"=w557) -> ("error out"=w552:errorcluster, "MotorControlDevRef"=w554:T9)  [unwired: 6 in, 1 out]
      n248 = call "Time Delay14"("error in (no error)"=w559, "Delay Time (s)"=1.0) -> ("error out"=w558:errorcluster)  [unwired: 9 in]
      n249 = call "Time Delay16"("error in (no error)"=w552, "Delay Time (s)"=1.0) -> ("error out"=w553:errorcluster)  [unwired: 9 in]
      n250 = call-poly <vilib>:"WPI_RobotDriveHolonomicDrive.vi"("Rotation"=0.0, "Direction"=0.0 ("X axis value"), "Magnitude"=0.0 ("X axis value"), "RobotDriveDevRef"=w591) -> ("Motor Values"=w596:dbl[])  [unwired: 5 in, 2 out]
      n251 = call-poly <vilib>:"SD Write Value.vi"("Numeric Array"=w596, "Name"=w565) -> ()  [unwired: 8 in, 2 out]
      n252 = call <vilib>:"WPI_MotorControlSetOutput.vi"("error in (no error)"=w558, "Output"=0.0, "MotorControlDevRef"=w562) -> ()  [unwired: 6 in, 3 out]
      n253 = call <vilib>:"WPI_MotorControlSetOutput.vi"("error in (no error)"=w553, "Output"=0.0, "MotorControlDevRef"=w554) -> ()  [unwired: 6 in, 3 out]
      n254 = call-poly <vilib>:"SD Write Value.vi"("Numeric Array"=w596, "Name"=w565) -> ()  [unwired: 8 in, 2 out]
    }
    frame Enabled {
    }
  }
  n255 = disable-structure shown="Disabled" {
    frame Enabled {
      n256 = call <vilib>:"WPI_AccelerometerRefNum Registry Get.vi"("refnum name"="Accel") -> ("error out"=w637:errorcluster, "AccelerometerDevRef"=w638:T21)  [unwired: 9 in]
      n257 = call <vilib>:"WPI_AccelerometerGetAcceleration.vi"("error in"=w637, "AccelerometerDevRef"=w638) -> ("Accelerations"=w636:T27)  [unwired: 7 in, 2 out]
      n258 = call <vilib>:"WPI_GyroRefNum Registry Get.vi"("refnum name"="Gyro") -> ("error out"=w627:errorcluster, "GyroDevRef"=w626:T16)  [unwired: 9 in]
      n259 = call <vilib>:"WPI_GyroGetAngle.vi"("error in"=w627, "GyroDevRef"=w626) -> ("Angle"=w623:dbl)  [unwired: 5 in, 4 out]
      n260 = Unbundle By Name(w636) -> ("X-Axis"=w625:dbl, "Y-Axis"=w624:dbl)
      n261 = call-poly <vilib>:"2D Cartesian Coordinate Rotation.vi"("theta"=w623, "y"=w624, "x"=w625) -> ("y out"=w621:dbl, "x out"=w622:dbl)  [unwired: 6 in, 1 out]
      n262 = feedback #1() -> (w634:dbl)  [unwired: 1 in]
      n263 = Add(x=w634, y=w622) -> (x+y=w619:dbl)
      n264 = feedback-in #1(w619) -> ()
      n265 = feedback #2() -> (w633:dbl)  [unwired: 1 in]
      n266 = Add(x=w621, y=w633) -> (x+y=w620:dbl)
      n267 = feedback-in #2(w620) -> ()
      n268 = Bundle(w619, w620) -> (w618:cluster{dbl, dbl})  [unwired: 1 in]
      n269 = feedback #3() -> (w629:dbl[])  [unwired: 1 in]
      n270 = feedback #4() -> (w631:dbl[])  [unwired: 1 in]
      n271 = call-poly <vilib>:"2D Cartesian Coordinate Shift.vi"("shift"=w618, "Y"=w629, "X"=w631) -> ("Y Out"=w630:dbl[], "X Out"=w632:dbl[])  [unwired: 6 in, 1 out]
      "X Out" <- w632
      "Y Out" <- w630
      n272 = feedback-in #3(w630) -> ()
      n273 = feedback-in #4(w632) -> ()
    }
    frame Disabled {
      # "Positioning System"
    }
  }
  n274 = disable-structure shown="Disabled" {
    frame Enabled {
    }
    frame Disabled {
      n275 = call <vilib>:"WPI_MotorControlRefNum Registry Get.vi"("refnum name"="Lift Motor 1") -> ()  [unwired: 9 in, 2 out]
      n276 = call <vilib>:"WPI_RobotDriveRefNum Registry Get.vi"("refnum name"="Intake") -> ()  [unwired: 9 in, 2 out]
      n277 = call <vilib>:"WPI_RobotDriveRefNum Registry Get.vi"("refnum name"="Four Motors") -> ()  [unwired: 9 in, 2 out]
      n278 = case shown="True" FALSE {
        frame False {
        }
        frame True {
        }
      }
    }
  }
